vi "Open FPGA Reference.vi"(8 "error in (no error)":errorcluster, 10 "Resource Name":T1, 11 "Data in":T2) -> (0 "error out":errorcluster, 3 "Data out":T2)   [LabVIEW 2017, in "Test Bench.lvlib"]
uses:
  Test Bench.lvlib
  Scan Engine Variables.ctl
  <instrlib>/_niInstr/FIFO Register Bus/v1/Host/niInstr FIFO Register Bus v1 Host.lvclass
  C:/Program Files (x86)/National Instruments/LabVIEW 2017/instr.lib/_niInstr/Instruction Framework/v1/Host/Instruction Target/niInstr Instruction Target v1 Host.lvclass
  <instrlib>/_niInstr/Instruction Framework/v1/Host/Instruction Framework Context/niInstr Instruction Framework Context v1 Host.lvclass
  <vilib>/userdefined/High Color/nirio_resource_hc.ctl
  <vilib>/FPGAPlugInAG/PCIe-7852R/niLvFpga_Open_PCIe-7852R.vi
  <vilib>/rvi/interface/common/dynamic/niFpgaDynamicAddResources.vi
  <instrlib>/_niInstr/Instruction Framework/v1/Host/Subsystem Map/Private/Lookup Single Context.vi
  <vilib>/rvi/interface/nirviOpenFPGA/nirviOpenFPGA.xnode
  FPGA Bitfiles/PCIe-7852R_Full.lvbitx
  <instrlib>/_niInstr/Instruction Framework/v1/Host/Subsystem Map/niInstr Subsystem Map v1 Host.lvclass
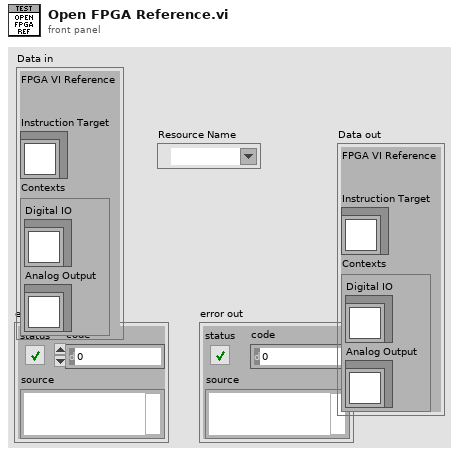
[diagram p1: front panel]
types:
  T1 = typedef "nirio_resource_hc.ctl" = tag
  T2 = typedef "Test Bench.lvlib/Scan Engine Variables.ctl" = cluster{"FPGA VI Reference":refnum<k20>, "Instruction Target":refnum<class "niInstr FIFO Register Bus v1 Host.lvclass">, "Contexts":cluster{"Digital IO":refnum<class "niInstr Instruction Framework Context v1 Host.lvclass">, "Analog Output":refnum<class "niInstr Instruction Framework Context v1 Host.lvclass">}}
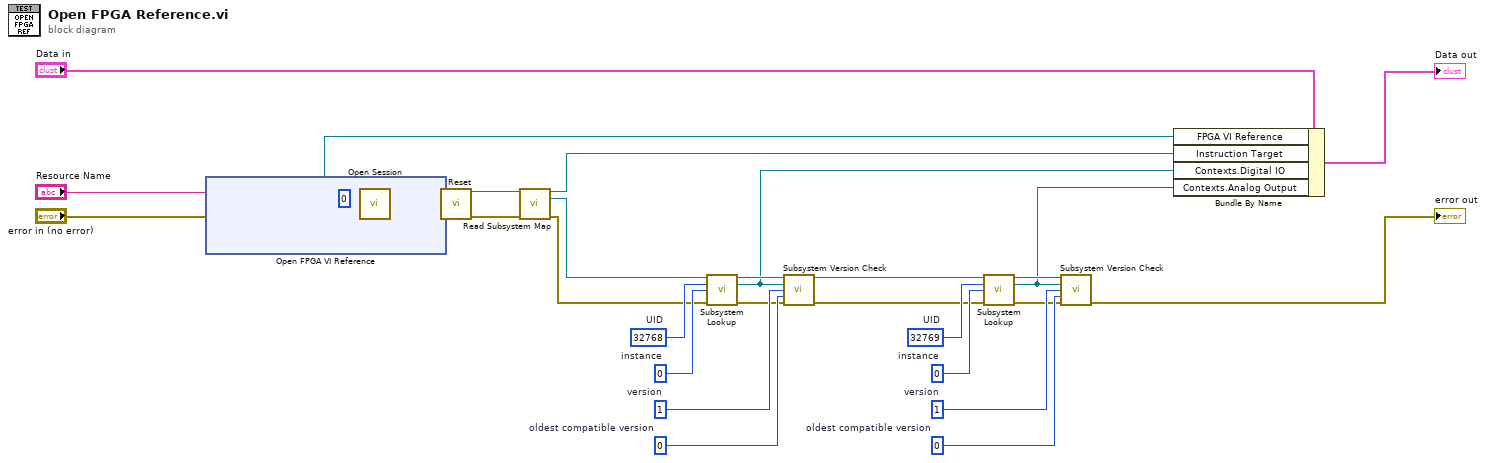
[diagram p0: block diagram]
diagram:
  w11 = u16 0  # oldest compatible version
  w10 = u16 1  # version
  w7 = u8 0  # instance
  w6 = u16 32769  # UID
  w19 = u16 0  # oldest compatible version
  w18 = u16 1  # version
  w15 = u8 0  # instance
  w14 = u16 32768  # UID
  n1 = xnode "Open FPGA VI Reference"("error in"="error in (no error)", "resource name"="Resource Name") -> ("FPGA VI Reference Out"=w23:refnum<k20>, "error out"=w27:errorcluster)
  n2 = call <instrlib>:"Open Session.vi"("fpga ref"=w23, "bus instance"=u32 0, "error in"=w27) -> ("session out"=w29:refnum<class "niInstr FIFO Register Bus v1 Host.lvclass">, "error out"=w28:errorcluster)  [unwired: 11 in]
  n3 = call-dynamic "Reset.vi"("session in"=w29, "error in"=w28) -> ("session out"=w31:refnum<class "niInstr FIFO Register Bus v1 Host.lvclass">, "error out"=w30:errorcluster)  [unwired: 12 in]
  n4 = call <instrlib>:"Read Subsystem Map.vi"("instruction target in"=w31, "error in"=w30) -> ("instruction target out"=w22:refnum<class "niInstr FIFO Register Bus v1 Host.lvclass">, "subsystem map"=w13:refnum<class "niInstr Subsystem Map v1 Host.lvclass">, "error out"=w2:errorcluster)  [unwired: 11 in]
  n5 = call-poly <instrlib>:"Subsystem Lookup.vi"("subsystem map in"=w13, "UID"=w14, "instance"=w15, "error in"=w2) -> ("subsystem map out"=w17:refnum<class "niInstr Subsystem Map v1 Host.lvclass">, "context"=w12:refnum<class "niInstr Instruction Framework Context v1 Host.lvclass">, "error out"=w16:errorcluster)  [unwired: 8 in, 1 out]
  n6 = call-dynamic "Subsystem Version Check.vi"("subsystem map in"=w17, "context"=w12, "version"=w18, "oldest compatible version"=w19, "error in"=w16) -> ("subsystem map out"=w5:refnum<class "niInstr Subsystem Map v1 Host.lvclass">, "error out"=w4:errorcluster)  [unwired: 7 in, 2 out]
  n7 = call-poly <instrlib>:"Subsystem Lookup.vi"("subsystem map in"=w5, "UID"=w6, "instance"=w7, "error in"=w4) -> ("subsystem map out"=w9:refnum<class "niInstr Subsystem Map v1 Host.lvclass">, "context"=w3:refnum<class "niInstr Instruction Framework Context v1 Host.lvclass">, "error out"=w8:errorcluster)  [unwired: 8 in, 1 out]
  n8 = call-dynamic "Subsystem Version Check.vi"("subsystem map in"=w9, "context"=w3, "version"=w10, "oldest compatible version"=w11, "error in"=w8) -> ("error out"=→"error out":errorcluster)  [unwired: 7 in, 3 out]
  n9 = Bundle By Name(cluster="Data in", "FPGA VI Reference"=w23, "Instruction Target"=w22, "Contexts.Digital IO"=w12, "Contexts.Analog Output"=w3) -> (→"Data out":T2)
